vi "Rinocloud_pagination_button_state.vi"(9 "previous refnum":refnum<vi>, 10 "next refnum":refnum<vi>, 11 "pagination parameters in":T1={"limit"=15.0, "total"=0.0, "offset"=0.0, "count"=0.0}) -> (3 "pagination info":string)   [LabVIEW 2013]
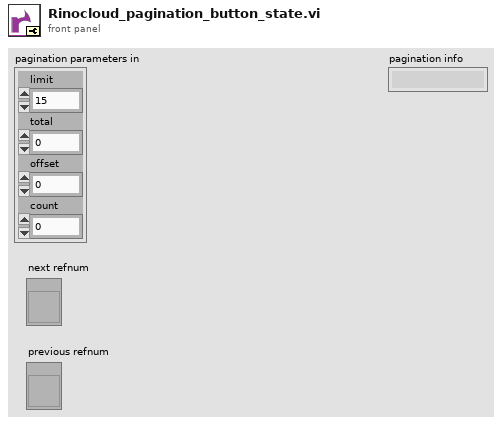
[diagram p1: front panel]
types:
  T1 = cluster{"limit":dbl, "total":dbl, "offset":dbl, "count":dbl}
  T2 = enum8{"Enabled", "Disabled", "Disabled and Grayed Out"}
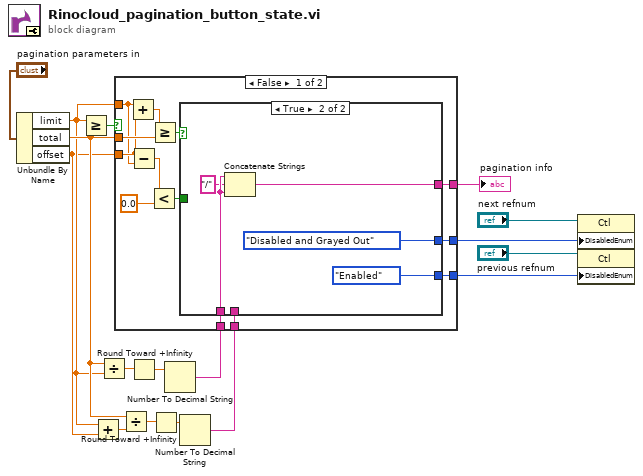
[diagram p0: block diagram]
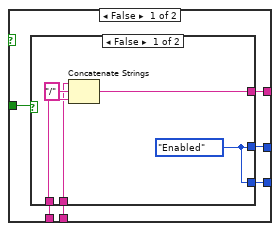
[diagram p2: hidden frame]
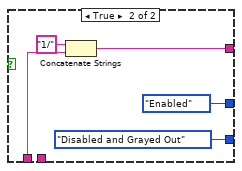
[diagram p3: hidden frame]
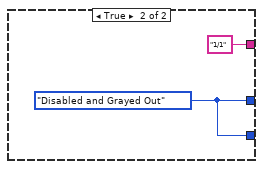
[diagram p4: hidden frame]
diagram:
  n1 = Unbundle By Name("pagination parameters in") -> ("limit"=w3:dbl, "total"=w5:dbl, "offset"=w2:dbl)
  n2 = Greater Or Equal?(x=w3, y=w5) -> (x >= y?=w16:bool)
  n3 = Add(x=w3, y=w2) -> (x+y=w4:dbl)
  n4 = Divide(x=w5, y=w3) -> (x/y=w10:dbl)
  n5 = Divide(x=w5, y=w4) -> (x/y=w6:dbl)
  n6 = Round Toward +Infinity(x=w10) -> (ceil(x): smallest int >= x=w9:dbl)
  n7 = Round Toward +Infinity(x=w6) -> (ceil(x): smallest int >= x=w7:dbl)
  n8 = Number To Decimal String(number=w9) -> (decimal integer string=w8:string)  [unwired: 1 in]
  n9 = Number To Decimal String(number=w7) -> (decimal integer string=w1:string)  [unwired: 1 in]
  n10 = case shown="False" w16 {
    tunnel: [w19 "1/1"] -> w15
    tunnel: w3 -> [w24 _]
    tunnel: w2 -> [w25 _]
    tunnel: w5 -> [w29 _]
    tunnel: [w27 w52] -> w14
    tunnel: [w26 w52] -> w13
    tunnel: w8 -> [w20 _]
    tunnel: w1 -> [w18 _]
    frame False {
      n11 = Add(x=w24, y=w25) -> (x+y=w30:dbl)
      n12 = Subtract(x=w25, y=w24) -> (x-y=w23:dbl)
      n13 = Less?(x=w23, y=0.0) -> (x < y?=w21:bool)
      n14 = Greater Or Equal?(x=w30, y=w29) -> (x >= y?=w28:bool)
      n15 = case shown="True" w28 {
        tunnel: [w34 T2."Disabled and Grayed Out" ("Disabled")] -> w27
        tunnel: [w35 T2."Enabled" ("Disabled")] -> w26
        tunnel: w21 -> [w36 _]
        tunnel: w20 -> [w33 w49]
        tunnel: [w32 w47] -> w19
        tunnel: w18 -> [w31 _]
        frame False {
          n16 = case shown="False" w36 {
            tunnel: [w41 T2."Disabled and Grayed Out" ("Disabled")] -> w35
            tunnel: [w41 T2."Enabled" ("Disabled")] -> w34
            tunnel: w33 -> [w39 w43]
            tunnel: [w37 w42] -> w32
            tunnel: w31 -> [w38 _]
            frame False {
              w41 = T2."Enabled" ("Disabled")
              n17 = Concatenate Strings(w38, "/" ("string"), w39) -> (w37:string)
            }
            frame True {
              n18 = Concatenate Strings("1/" ("string"), w43) -> (w42:string)
            }
          }
        }
        frame True {
          n19 = Concatenate Strings(w49, "/" ("string"), w49) -> (w47:string)
        }
      }
    }
    frame True {
      w52 = T2."Disabled and Grayed Out" ("Disabled")
    }
  }
  "pagination info" <- w15
  n20 = property class="Ctl"(reference="next refnum", "DisabledEnum"=w14) -> ()  [unwired: 1 in, 2 out]
  n21 = property class="Ctl"(reference="previous refnum", "DisabledEnum"=w13) -> ()  [unwired: 1 in, 2 out]
